vi "Set VI Ref.vi"(1 "Instrument Prop In":T1={"Public"={"Column Name"=[], "Trace Color"=[]}, "Private"={"Path"=path "", "VI Refnum"=refnum, "Name"="", "# of Values"=0, "Scale Factors"=[], "Display"=[], "Offset"=[1.0]}} {"Private"."Offset" format="%^_3e"; "Private"."Scale Factors" format="%^_3e"}) -> (0 "Instrument Prop Out":T1={"Public"={"Column Name"=[], "Trace Color"=[]}, "Private"={"Path"=path "", "VI Refnum"=refnum, "Name"="", "# of Values"=0, "Scale Factors"=[], "Display"=[], "Offset"=[1.0]}} {"Private"."Offset" format="%^_3e"; "Private"."Scale Factors" format="%^_3e"})   [LabVIEW 2020]
uses:
  Sub Controls/Instrument Properties.ctl
  Sub Controls/Public.ctl
  Sub Controls/Private.ctl
  Sub Controls/Instrument Ref.ctl
  Sub Controls/SystemCheckBox-resize.ctl
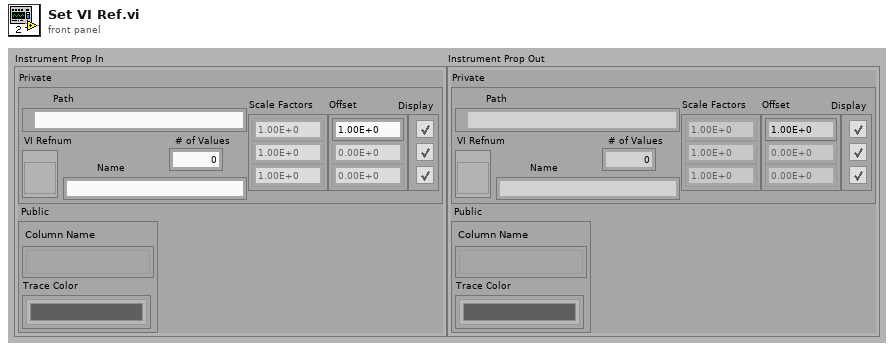
[diagram p1: front panel]
types:
  T1 = typedef "Instrument Properties.ctl" = cluster{"Public":T2, "Private":T3}
  T2 = typedef "Public.ctl" = cluster{"Column Name":string[], "Trace Color":u32[]}
  T3 = typedef "Private.ctl" = cluster{"Path":path, "VI Refnum":T4, "Name":string, "# of Values":i32, "Scale Factors":dbl[], "Display":T5[], "Offset":dbl[]}
  T4 = typedef "Instrument Ref.ctl" = refnum<vi>
  T5 = typedef "SystemCheckBox-resize.ctl" = bool
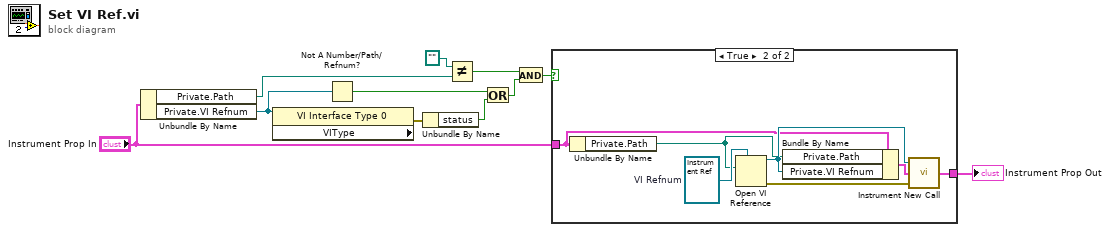
[diagram p0: block diagram]
diagram:
  n1 = Unbundle By Name("Instrument Prop In") -> ("Private.Path"=w4:path, "Private.VI Refnum"=w8:T4)
  n2 = property class="VI Interface Type 0" props=["VIType"](reference=w8) -> (error out=w6:errorcluster)  [unwired: 1 in, 2 out]
  n3 = Not A Number/Path/Refnum?(number/path/refnum=w8) -> (NaN/Path/Refnum?=w9:bool)
  n4 = Unbundle By Name(w6) -> ("status"=w5:bool)
  n5 = Not Equal?(x=path "", y=w4) -> (x != y?=w1:bool)
  n6 = Or(x=w9, y=w5) -> (x .or. y?=w7:bool)
  n7 = And(x=w1, y=w7) -> (x .and. y?=w2:bool)
  n8 = case shown="True" w2 {
    tunnel: "Instrument Prop In" -> [w12 w16]
    tunnel: [w12 w14] -> w10
    frame False {
    }
    frame True {
      w19 = T4 refnum  # VI Refnum
      n9 = Unbundle By Name(w16) -> ("Private.Path"=w13:path)
      n10 = Open VI Reference(type specifier VI Refnum (for type only)=w19, vi path=w13) -> (vi reference=w18:T4, error out=w17:errorcluster)  [unwired: 4 in]
      n11 = Bundle By Name(cluster=w16, "Private.Path"=w13, "Private.VI Refnum"=w18) -> (w15:T1)
      n12 = call "Instrument New Call.vi"("Error In"=w17, "Instrument Prop In"=w15, "VI Refnum"=w18) -> ("Instrument Prop Out"=w14:T1)  [unwired: 1 in, 1 out]
    }
  }
  "Instrument Prop Out" <- w10
